vi "Stop  LV2.vi"(0 "Operation":T1, 5 "Stop":bool, 11 "Error in":errorcluster) -> (4 "Output":bool, 15 "Error out":errorcluster)   [LabVIEW 2020]
doc: "This VI is used as a LV2 global to store and retrive boolean input between different VIs"
uses:
  Assignment backups/Assignment07 1/Assignment07/Generate and Acquire/Typedefs/Stop cases.ctl
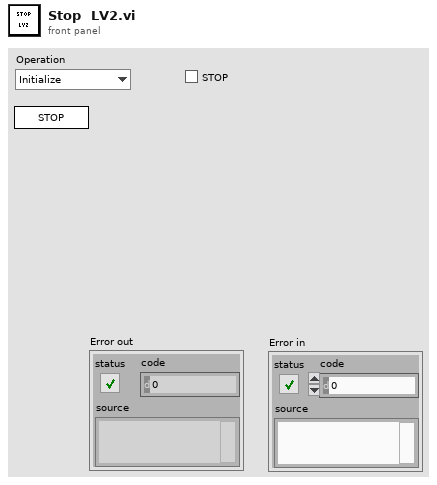
[diagram p1: front panel]
types:
  T1 = typedef "Stop cases.ctl" = enum16{"Initialize", "Write", "Stop"}
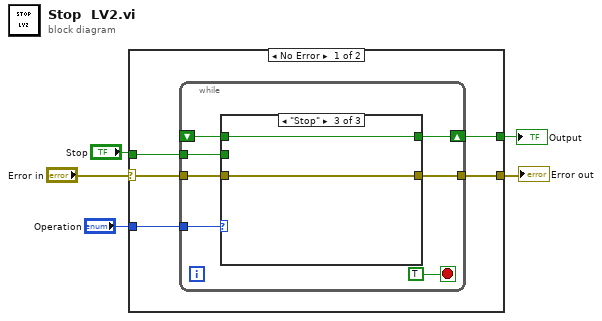
[diagram p0: block diagram]
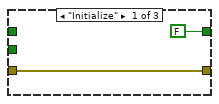
[diagram p2: hidden frame]
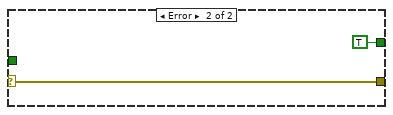
[diagram p4: hidden frame]
diagram:
  n1 = case shown="No Error" "Error in" {
    selector: "Error in" -> [w8 w25]
    tunnel: "Operation" -> [w10 _]
    tunnel: "Stop" -> [w9 _]
    tunnel: [w7 w25] -> w2
    tunnel: [w6 TRUE ("Stop")] -> w1
    frame No Error {
      n2 = while {
        tunnel: w10 -> [w17]
        shift-right: [w16] -> w6
        shift-left: _ -> [w14]
        tunnel: w9 -> [w15]
        tunnel: w8 -> [w12]
        tunnel: [w11] -> w7
        stop <- TRUE stop-if-true
        n3 = case shown="\"Stop\"" w17 {
          tunnel: [FALSE w21 w23] -> w16
          tunnel: w15 -> [_ w21 _]
          tunnel: w14 -> [_ _ w23]
          tunnel: w12 -> [w19 w20 w22]
          tunnel: [w19 w20 w22] -> w11
          frame "Initialize" {
          }
          frame "Write" {
          }
          frame "Stop" {
          }
        }
      }
    }
    frame Error {
    }
  }
  "Output" <- w1
  "Error out" <- w2
